vi "SetSampleRate.vi"(4 "TimeBase":cluster{"Time/Div":dbl}={"Time/Div"=5e-06} {"Time/Div" scale=5e-06..0.2}, 6 "Channel Setting 1":T1={"physical channels"="", "Enable"=FALSE, "Coupling"=enum."DC", "    Scale\n  Volts/Div  "=0.01, "    Vertical\nPosition (Div)"=0.0, "Meas Range"=0.1} {"Meas Range" items=["-0.1 V~+0.1 V"=0.1, "-0.2 V~0.2 V"=0.2, "-0.5 V~+0.5 V"=0.5, "-1 V~+1 V"=1.0, "-2 V~+2 V"=2.0, "-5 V~+5 V"=5.0, "-10 V~+10 V"=10.0]; "Vertical\nPosition (Div)" min=-5.0 max=5.0 step=0.01 scale=-5.0..5.0 scale format="%.2f"; "Scale\n  Volts/Div" scale=0.01..20.0}, 7 "Error In":errorcluster caption="错误输入", 8 "Task In":refnum<k21> caption="任务输入", 9 "Channel Setting 0":T1={"physical channels"="", "Enable"=FALSE, "Coupling"=enum."DC", "    Scale\n  Volts/Div  "=0.01, "    Vertical\nPosition (Div)"=0.0, "Meas Range"=0.1} {"Meas Range" items=["-0.1 V~+0.1 V"=0.1, "-0.2 V~0.2 V"=0.2, "-0.5 V~+0.5 V"=0.5, "-1 V~+1 V"=1.0, "-2 V~+2 V"=2.0, "-5 V~+5 V"=5.0, "-10 V~+10 V"=10.0]; "Vertical\nPosition (Div)" min=-5.0 max=5.0 step=0.01 scale=-5.0..5.0 scale format="%.2f"; "Scale\n  Volts/Div" scale=0.01..20.0}) -> (0 "采样率":string, 1 "Error Out":errorcluster caption="错误输出", 3 "Task Out":refnum<k21> caption="任务输出")   [LabVIEW 2012]
uses:
  GlobalVariable.vi
  <vilib>/DAQmx/configure/timing.llb/DAQmx Timing (Sample Clock).vi
  <resource>/objmgr/daqmx.rc
panel:
  # "Channel 1 Settings"
  # "Channel 0 Settings"
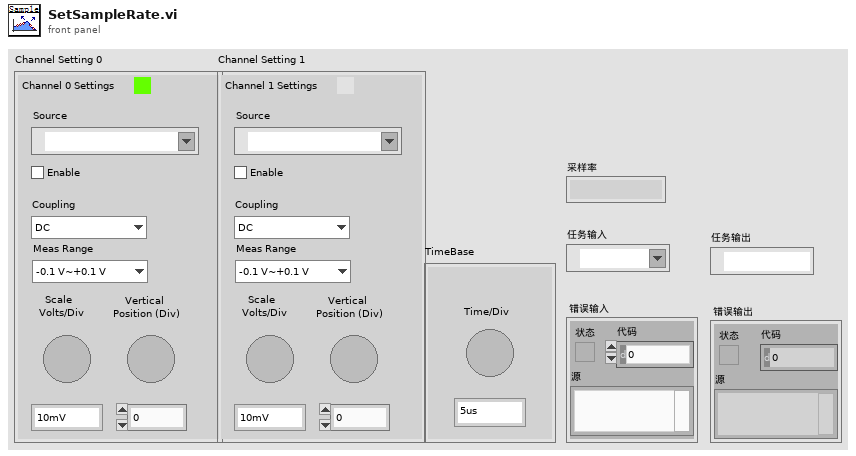
[diagram p1: front panel]
types:
  T1 = cluster{"physical channels":tag, "Enable":bool, "Coupling":enum16{"DC", "AC"}, "    Scale\n  Volts/Div  ":dbl, "    Vertical\nPosition (Div)":dbl, "Meas Range":dbl}
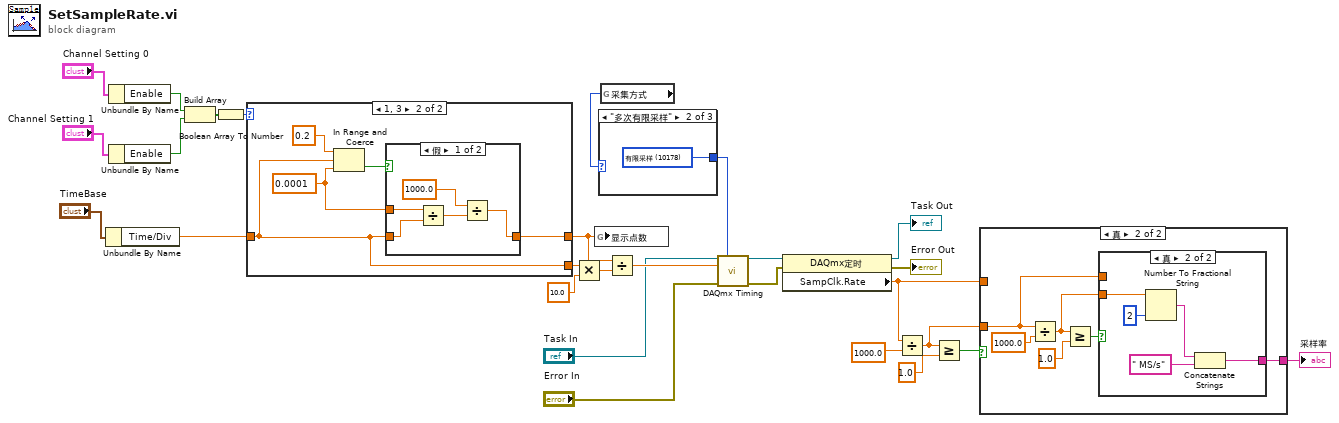
[diagram p0: block diagram]
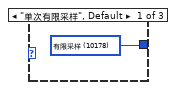
[diagram p2: hidden frame]
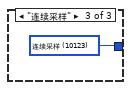
[diagram p3: hidden frame]
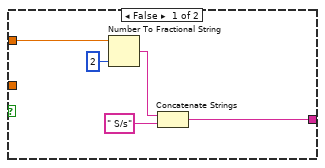
[diagram p4: hidden frame]
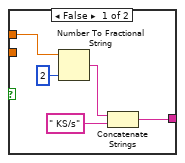
[diagram p5: hidden frame]
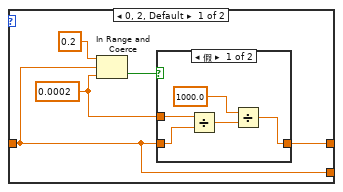
[diagram p6: hidden frame]
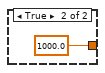
[diagram p7: hidden frame]
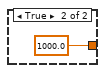
[diagram p8: hidden frame]
diagram:
  n1 = Unbundle By Name("TimeBase") -> ("Time/Div"=w12:dbl)
  n2 = Unbundle By Name("Channel Setting 0") -> ("Enable"=w24:bool)
  n3 = Unbundle By Name("Channel Setting 1") -> ("Enable"=w23:bool)
  n4 = Build Array(w24, w23) -> (w27:bool[])
  n5 = Boolean Array To Number(Boolean array=w27) -> (number=w22:u32)
  n6 = case shown="1, 3" w22 {
    tunnel: w12 -> [w28 w39]
    tunnel: [w29 w40] -> w8
    tunnel: [w28 w39] -> w11
    frame 0, 2, Default {
      w30 = 0.0002 ("下限")
      n7 = In Range and Coerce(upper limit=0.2 ("上限"), x=w28, lower limit=w30) -> (In Range?=w31:bool)  [unwired: 1 out]
      n8 = case shown="假" w31 {
        tunnel: w28 -> [w36 _]
        tunnel: [w33 1000.0] -> w29
        tunnel: w30 -> [w37 _]
        frame False {
          n9 = Divide(x=w37, y=w36) -> (x/y=w35:dbl)
          n10 = Divide(x=1000.0, y=w35) -> (x/y=w33:dbl)
        }
        frame True {
        }
      }
    }
    frame 1, 3 {
      w43 = 0.0001 ("下限")
      n11 = In Range and Coerce(upper limit=0.2 ("上限"), x=w39, lower limit=w43) -> (In Range?=w42:bool)  [unwired: 1 out]
      n12 = case shown="假" w42 {
        tunnel: w39 -> [w47 _]
        tunnel: [w44 1000.0] -> w40
        tunnel: w43 -> [w48 _]
        frame False {
          n13 = Divide(x=w48, y=w47) -> (x/y=w46:dbl)
          n14 = Divide(x=1000.0, y=w46) -> (x/y=w44:dbl)
        }
        frame True {
        }
      }
    }
  }
  n15 = Multiply(x=w11, y=10.0) -> (x*y=w9:dbl)
  n16 = global write "GlobalVariable.vi" "显示点数"(w8) -> ()
  n17 = global read "GlobalVariable.vi" "采集方式"() -> (w2:enum16{"单次有限采样", "多次有限采样", "连续采样"})
  n18 = case shown="\"多次有限采样\"" w2 {
    tunnel: [w50 w51 w52] -> w1
    frame "单次有限采样", Default {
      w50 = 10178 items=["有限采样"=10178, "连续采样"=10123, "硬件定时单点"=12522] ("sample mode")
    }
    frame "多次有限采样" {
      w51 = 10178 items=["有限采样"=10178, "连续采样"=10123, "硬件定时单点"=12522] ("sample mode")
    }
    frame "连续采样" {
      w52 = 10123 items=["有限采样"=10178, "连续采样"=10123, "硬件定时单点"=12522] ("sample mode")
    }
  }
  n19 = Divide(x=w8, y=w9) -> (x/y=w7:dbl)
  n20 = call-poly <vilib>:"DAQmx Timing.vi"("task/channels in"="Task In", "sample mode"=w1, "rate"=w7, "error in"="Error In") -> ("task out"=w4:refnum<k21>, "error out"=w3:errorcluster)  [unwired: 10 in]
  n21 = property class="DAQmx定时"(reference=w4, error in=w3) -> (reference out=→"Task Out":refnum<k21>, error out=→"Error Out":errorcluster, "SampClk.Rate"=w15:dbl)
  n22 = Divide(x=w15, y=1000.0) -> (x/y=w14:dbl)
  n23 = Greater Or Equal?(x=w14, y=1.0) -> (x >= y?=w17:bool)
  n24 = case shown="真" w17 {
    tunnel: w15 -> [w57 _]
    tunnel: [w54 w58] -> w13
    tunnel: w14 -> [_ w60]
    frame False {
      n25 = Number To Fractional String(number=w57, precision (6)=i16 2 ("精度(6)")) -> (F-format string=w56:string)  [unwired: 2 in]
      n26 = Concatenate Strings(w56, " S/s" ("字符串")) -> (w54:string)
    }
    frame True {
      n27 = Divide(x=w60, y=1000.0) -> (x/y=w59:dbl)
      n28 = Greater Or Equal?(x=w59, y=1.0) -> (x >= y?=w61:bool)
      n29 = case shown="真" w61 {
        tunnel: w60 -> [w65 _]
        tunnel: w59 -> [_ w70]
        tunnel: [w64 w69] -> w58
        frame False {
          n30 = Number To Fractional String(number=w65, precision (6)=i16 2 ("精度(6)")) -> (F-format string=w68:string)  [unwired: 2 in]
          n31 = Concatenate Strings(w68, " KS/s" ("字符串")) -> (w64:string)
        }
        frame True {
          n32 = Number To Fractional String(number=w70, precision (6)=i16 2 ("精度(6)")) -> (F-format string=w73:string)  [unwired: 2 in]
          n33 = Concatenate Strings(w73, " MS/s" ("字符串")) -> (w69:string)
        }
      }
    }
  }
  "采样率" <- w13
